vi "F5000_Find_V.vi"(8 "Error In":errorcluster, 11 "String in":string) -> (0 "Error Out":errorcluster, 3 "String out":string)   [LabVIEW 2018]
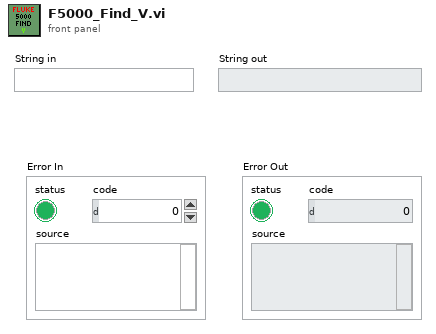
[diagram p1: front panel]
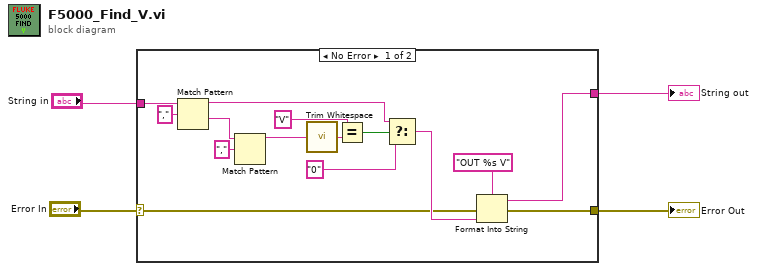
[diagram p0: block diagram]
diagram:
  n1 = case shown="No Error" "Error In" {
    selector: "Error In" -> [w5 w20]
    tunnel: "String in" -> [w19 _]
    tunnel: [w7 _] -> w1
    tunnel: [w6 w20] -> w4
    frame No Error {
      n2 = Match Pattern(string=w19, regular expression=",") -> (before substring=w16:string, after substring=w10:string)  [unwired: 1 in, 2 out]
      n3 = Match Pattern(string=w10, regular expression=",") -> (before substring=w12:string)  [unwired: 1 in, 3 out]
      n4 = call <vilib>:"Trim Whitespace.vi"("string"=w12) -> ("trimmed string"=w13:string)  [unwired: 1 in]
      n5 = Equal?(x="V", y=w13) -> (x = y?=w15:bool)
      n6 = Select(t=w16, s=w15, f="0") -> (s? t:f=w18:string)
      n7 = Format Into String(format string="OUT %s V", error in=w5, w18) -> (resulting string=w7:string, error out=w6:errorcluster)  [unwired: 1 in]
    }
    frame Error {
    }
  }
  "Error Out" <- w4
  "String out" <- w1
